vi "WriteTemplate.vi"(8 "error in":errorcluster, 10 "PropIn":bool=TRUE, 11 "ObjIn":refnum<class>) -> (0 "error out":errorcluster, 3 "ObjOut":refnum<class>)   [LabVIEW 2013]
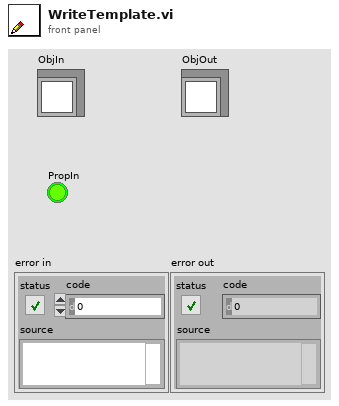
[diagram p1: front panel]
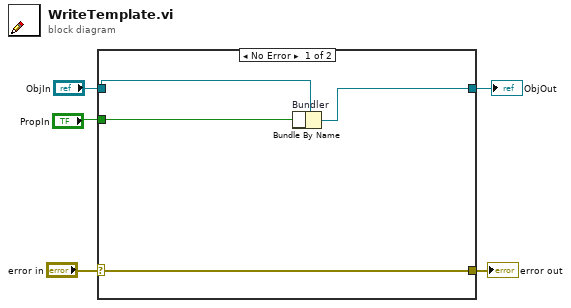
[diagram p0: block diagram]
diagram:
  n1 = case shown="No Error" "error in" {
    selector: "error in" -> [w9 w11]
    tunnel: "ObjIn" -> [w7 w10]
    tunnel: [w6 w10] -> w4
    tunnel: [w9 w11] -> w2
    tunnel: "PropIn" -> [w8 _]
    frame No Error {
      n2 = Bundle By Name "Bundler"(cluster=w7, w8) -> (w6:refnum<class>)
    }
    frame Error {
    }
  }
  "ObjOut" <- w4
  "error out" <- w2
